vi "FPGA ENCODER.vi"() -> ()   [LabVIEW 2017]
uses:
  <vilib>/rvi/Emulation/niFpgaGetClockAttributes.vi
  <vilib>/rvi/Emulation/niFpgaSctlEmulationGetInTimedLoop.vi
  <vilib>/rvi/Emulation/niFpgaEmulationReportErrorSimple.vi
  <vilib>/rvi/eio/common/nirviEmuTemplateMethod_errors.vi
  <vilib>/rvi/Emulation/niFpgaCriticalErrorInLSC.vi
  <vilib>/eio/EIONode/EIONode.xnode
panel:
  out "Direction":bool
  out "*2.5E-8 Second/Period":u32
  out "Pulses/Millisecond":i32
  out "ConnectorC/AI1":i16
  out "ConnectorC/AI0":i16
  in  "ConnectorC/AO1":i16
  in  "ConnectorC/AO0":i16
  in  "Debounce Ticks":u16=5
  out "CNTR":u32
  out "STAT":u8 format="%08b"
  in  "CNFG":u8 format="%08b"
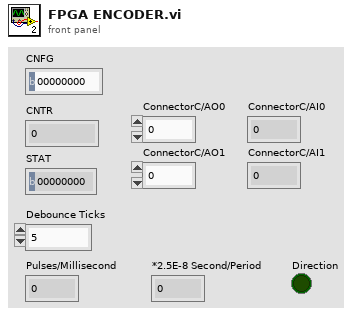
[diagram p1: front panel]
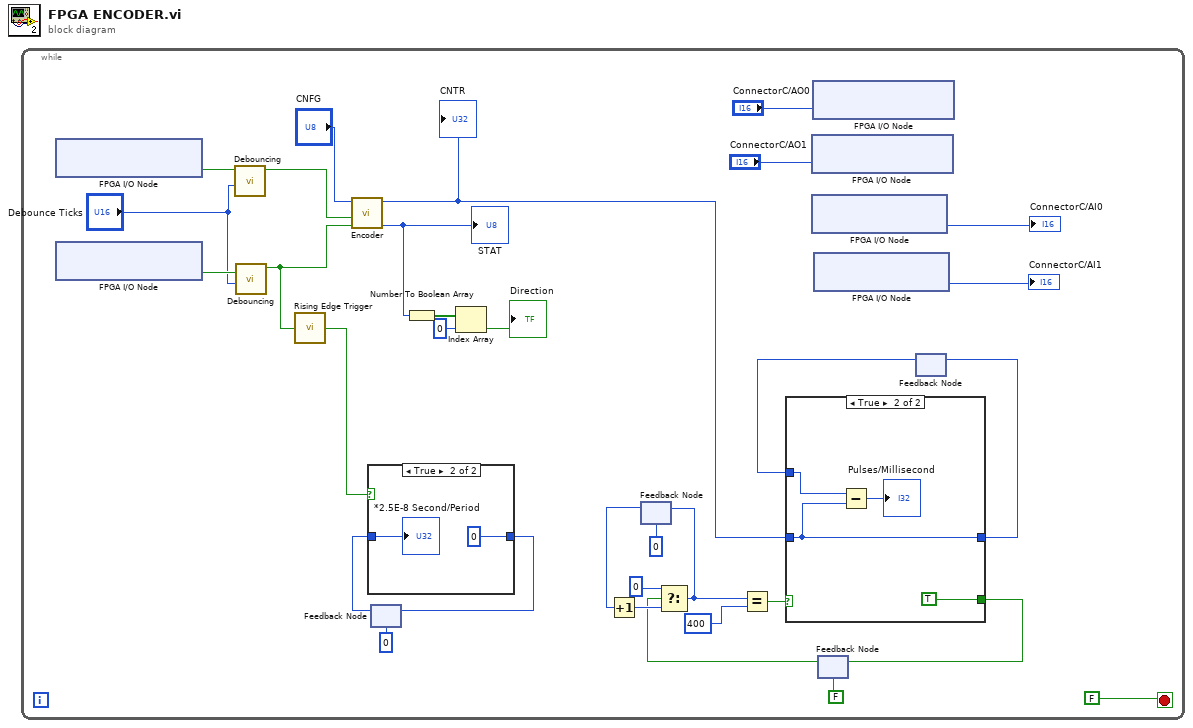
[diagram p0: block diagram]
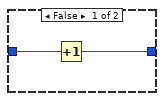
[diagram p2: hidden frame]
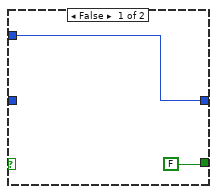
[diagram p3: hidden frame]
diagram:
  n1 = while {
    stop <- FALSE stop-if-true
    n2 = xnode "FPGA I/O Node"() -> ("ConnectorC/DIO1"=w32:bool)  [unwired: 1 in, 1 out]
    n3 = xnode "FPGA I/O Node"() -> ("ConnectorC/DIO3"=w31:bool)  [unwired: 1 in, 1 out]
    n4 = call "Debouncing.vi"("Debounce Ticks"="Debounce Ticks", "Input Signal"=w32) -> ("Debounced Signal"=w29:bool)  [unwired: 9 in]
    n5 = call "Debouncing.vi"("Debounce Ticks"="Debounce Ticks", "Input Signal"=w31) -> ("Debounced Signal"=w7:bool)  [unwired: 9 in]
    n6 = call "Rising Edge Trigger.vi"("Signal"=w7) -> ("Trigger?"=w4:bool)
    n7 = call "Encoder.vi"("Phase B"=w7, "Phase A"=w29, "CNFG"="CNFG") -> ("STAT"=w10:u8, "CNTR"=w11:u32)  [unwired: 7 in]
    "STAT" <- w10
    "CNTR" <- w11
    n8 = feedback #1(i16 0) -> (w5:i16)
    n9 = case shown="True" w4 {
      tunnel: [w34 i16 0] -> w6
      tunnel: w5 -> [w33 w35]
      frame False {
        n10 = Increment(x=w33) -> (x+1=w34:i16)
      }
      frame True {
        "*2.5E-8 Second/Period" <- w35
      }
    }
    n11 = feedback-in #1(w6) -> ()
    n12 = Number To Boolean Array(number=w10) -> (Boolean array=w9:bool[])
    n13 = Index Array(array=w9, index=0) -> (element=→"Direction":bool)
    n14 = feedback #2(u32 0 ("t")) -> (w21:u32)
    n15 = Increment(x=w21) -> (x+1=w22:u32)
    n16 = xnode "FPGA I/O Node"("ConnectorC/AO1"="ConnectorC/AO1") -> ()  [unwired: 1 in, 1 out]
    n17 = xnode "FPGA I/O Node"() -> ("ConnectorC/AI0"=→"ConnectorC/AI0":i16)  [unwired: 1 in, 1 out]
    n18 = xnode "FPGA I/O Node"("ConnectorC/AO0"="ConnectorC/AO0") -> ()  [unwired: 1 in, 1 out]
    n19 = xnode "FPGA I/O Node"() -> ("ConnectorC/AI1"=→"ConnectorC/AI1":i16)  [unwired: 1 in, 1 out]
    n20 = feedback #3(FALSE) -> (w15:bool)
    n21 = Select(t=u32 0, s=w15, f=w22) -> (s? t:f=w20:u32)
    n22 = feedback-in #2(w20) -> ()
    n23 = Equal?(x=w20, y=u32 400) -> (x = y?=w18:bool)
    n24 = feedback #4() -> (w12:u32)  [unwired: 1 in]
    n25 = case shown="True" w18 {
      tunnel: w11 -> [_ w40]
      tunnel: [FALSE TRUE] -> w16
      tunnel: [w37 w40] -> w13
      tunnel: w12 -> [w37 w41]
      frame False {
      }
      frame True {
        n26 = Subtract(x=w41, y=w40) -> (x-y=→"Pulses/Millisecond":u32)
      }
    }
    n27 = feedback-in #3(w16) -> ()
    n28 = feedback-in #4(w13) -> ()
  }
